vi "Actor Core.vi"(8 "error in":errorcluster, 11 "SPIController in":refnum<class "SPIController.lvclass">) -> (0 "error out":errorcluster, 3 "Actor out":refnum<class "Actor.lvclass">)   [LabVIEW 2023, in "SPIController.lvlib" / "SPIController.lvclass"]
doc: "(<B>Filename</B>: Actor Framework.lvlib:Actor.lvclass:Actor Core.vi)\n\nReceives messages to the actor, reacts to them, and initiates any error handling that may shut the actor down.\n\nDescendant classes may override this VI to append parallel tasks for the actor to complete while it handles messages. Overrides use the Call Parent Class Method node."
uses:
  SPIController.lvclass
  C:/Program Files/National Instruments/LabVIEW 2023/vi.lib/ActorFramework/Actor/Actor.lvclass
  <vilib>/ActorFramework/Actor/Actor.lvclass
  Controller_Cluster.ctl
  Controller_Scan_Cluster.ctl
  TranslationStage_UI/TranslationStage_UI/TranslationStageUI.lvclass
  <vilib>/ActorFramework/Message Enqueuer/Message Enqueuer.lvclass
  SinglePhotonInterferenceUI/SinglePhotonInterferenceUI/SinglePhotonInterferenceUI.lvclass
  <vilib>/ActorFramework/Actor/Actor.lvclass/Actor.ctl
  <vilib>/ActorFramework/Message Enqueuer/Message Enqueuer.lvclass/Message Enqueuer.ctl
  SPIController.lvclass/SPIController.ctl
  <vilib>/ActorFramework/Message Enqueuer/Init from Existing Queue.vi
  <vilib>/ActorFramework/Message Enqueuer/Enqueue.vi
  <vilib>/ActorFramework/Stop Msg/Stop Msg.lvclass
  C:/Program Files/National Instruments/LabVIEW 2023/vi.lib/ActorFramework/Message/Message.lvclass
  <vilib>/ActorFramework/Message Priority Queue/Priority Enqueue.vi
  SPIController.lvlib
  typedefs/typedefs.lvlib
panel:
  out "Multiharp Enqueuer":refnum<class "Message Enqueuer.lvclass">
  out "Translation Stage Enqueuer":refnum<class "Message Enqueuer.lvclass">
  out "Self Enqueuer":refnum<class "Message Enqueuer.lvclass">
  in  "TranslationStageUI.lvclass":refnum<class "TranslationStageUI.lvclass">
  in  "Ctrl Cluster":T1={"Actors Off"=FALSE, "Scan Cluster"={"Scan Segments X"=0, "Scan Segments Y"=0, "X Segments Left"=100, "Y Segments Left"=0, "Acq per step"=1, "X Home"=FALSE, "Y Home"=FALSE, "Axis"=enum."X", "Acquisitions Done"=0, "Get Measurements?"=FALSE}} {"Scan Cluster"."Scan Segments Y" max=100 step=1 scale=0.0..100.0; "Scan Cluster"."Acq per step" min=1 max=10000 step=1 scale=1.0..10000.0; "Scan Cluster"."Scan Segments X" max=100 step=1 scale=0.0..100.0}
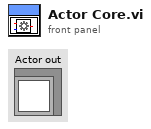
[diagram p1: front panel]
types:
  T1 = typedef "typedefs.lvlib/Controller_Cluster.ctl" = cluster{"Actors Off":bool, "Scan Cluster":T2}
  T2 = typedef "typedefs.lvlib/Controller_Scan_Cluster.ctl" = cluster{"Scan Segments X":u32, "Scan Segments Y":u32, "X Segments Left":u16, "Y Segments Left":u16, "Acq per step":u32, "X Home":bool, "Y Home":bool, "Axis":enum16{"X", "Y", "Z", "HOM"}, "Acquisitions Done":u16, "Get Measurements?":bool}
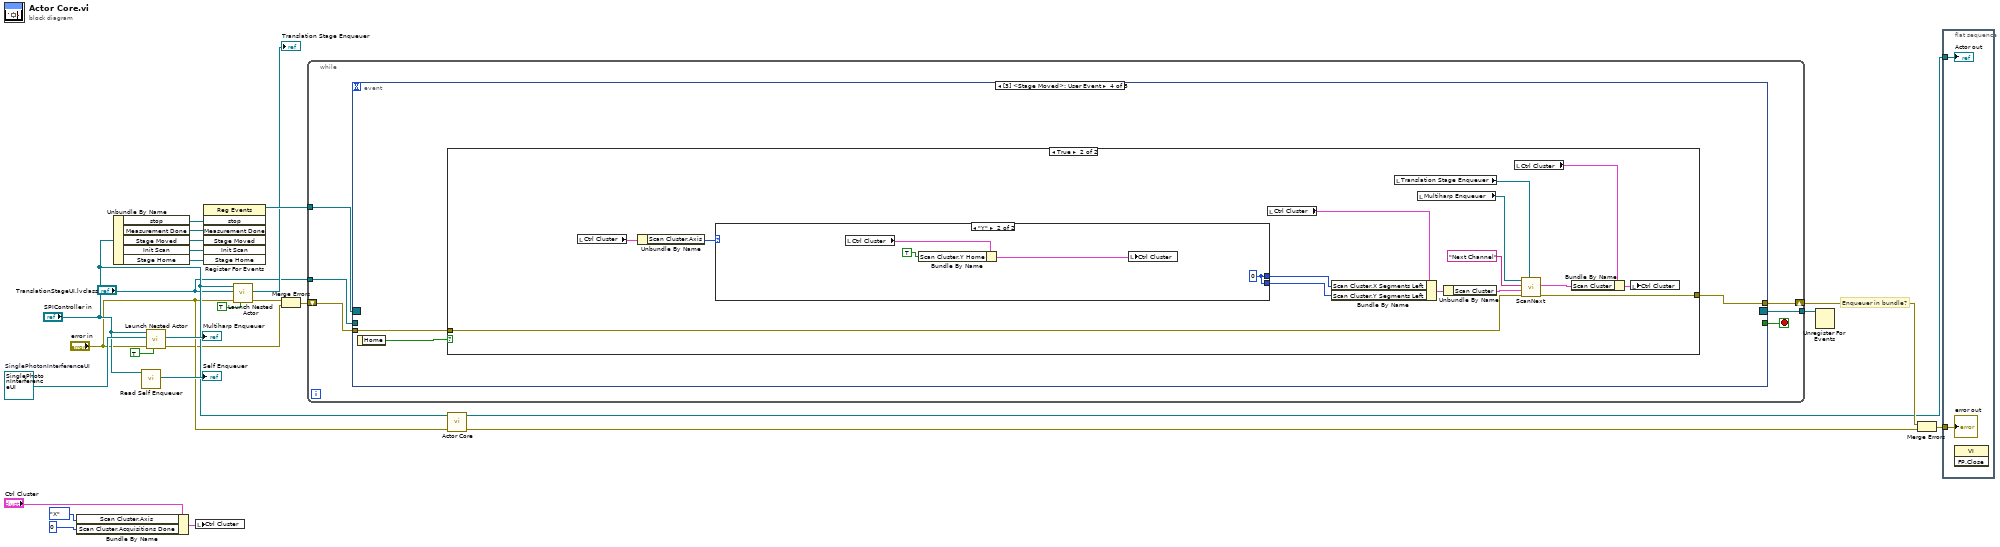
[diagram p0: block diagram]
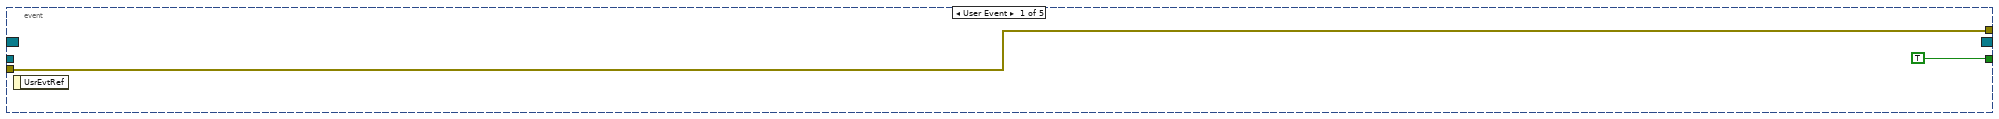
[diagram p2: hidden frame]
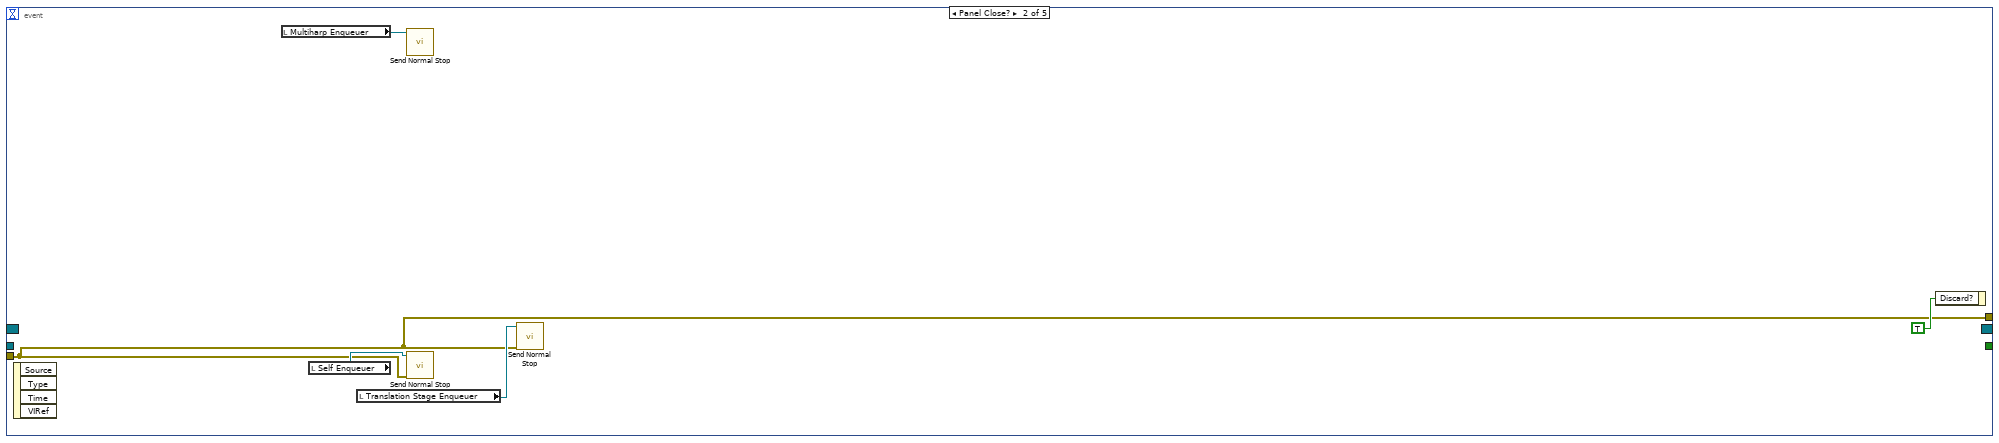
[diagram p3: hidden frame]
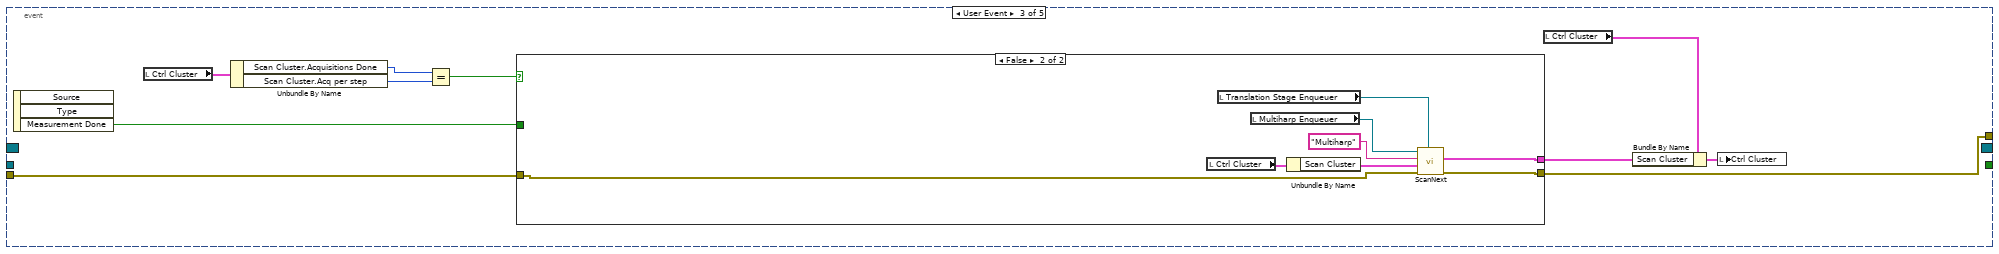
[diagram p4: hidden frame]
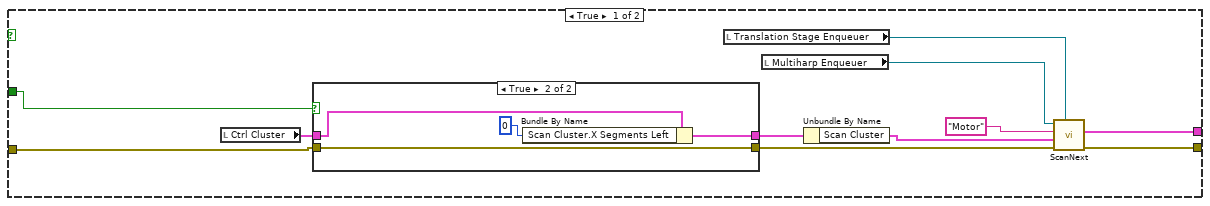
[diagram p5: hidden frame]
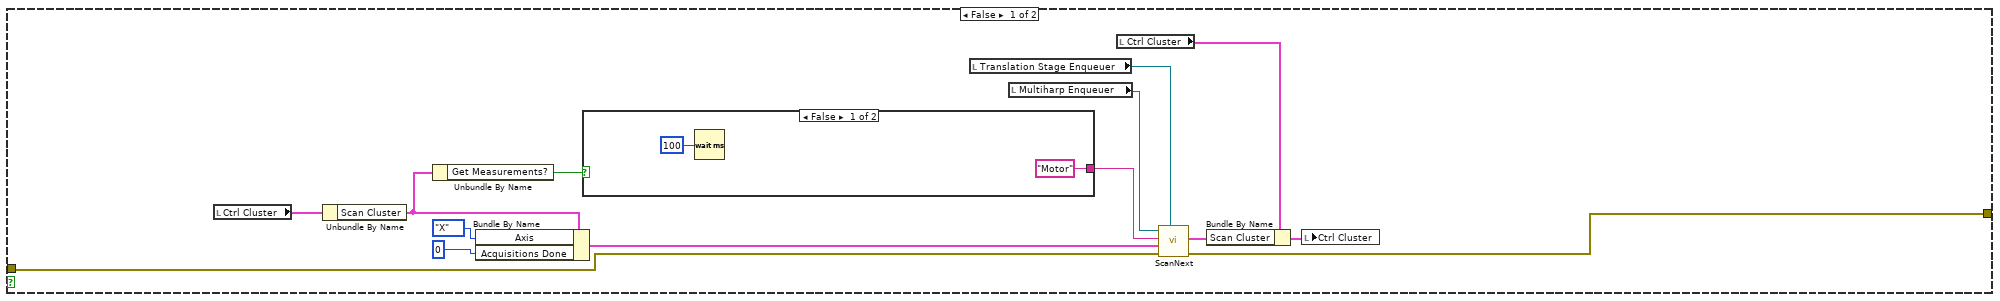
[diagram p7: hidden frame]
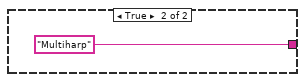
[diagram p8: hidden frame]
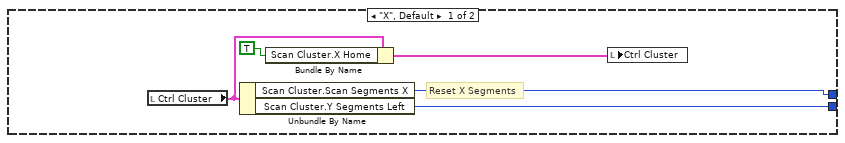
[diagram p9: hidden frame]
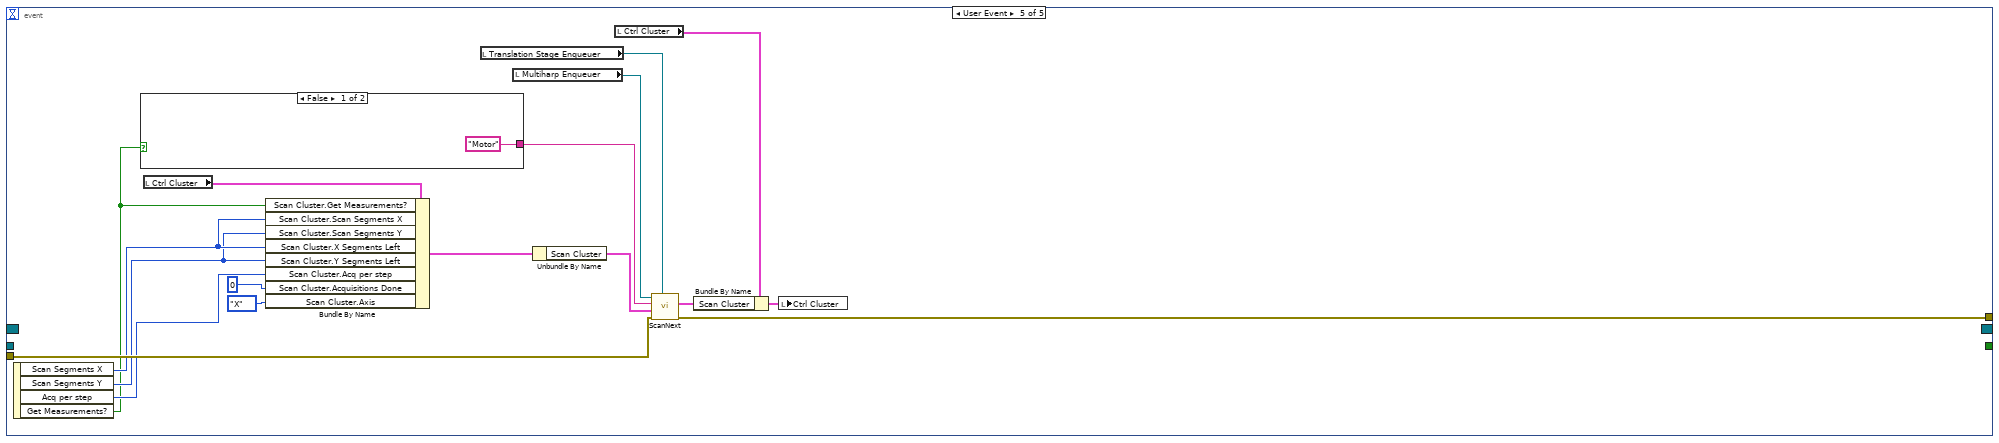
[diagram p10: hidden frame]
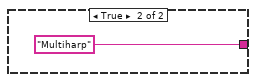
[diagram p11: hidden frame]
diagram:
  w27 = refnum<class "SinglePhotonInterferenceUI.lvclass"> refnum  # SinglePhotonInterferenceUI
  # "Enqueuer in bundle?"
  n1 = Bundle By Name(cluster="Ctrl Cluster", "Scan Cluster.Axis"=enum16{"X", "Y", "Z", "HOM"}."X", "Scan Cluster.Acquisitions Done"=u16 0) -> (w5:T1)
  n2 = Unbundle By Name("SPIController in") -> ("stop"=w24:refnum<user-event>, "Measurement Done"=w23:refnum<user-event>, "Stage Moved"=w15:refnum<user-event>, "Init Scan"=w14:refnum<user-event>, "Stage Home"=w13:refnum<user-event>)
  n3 = call <vilib>:"Read Self Enqueuer.vi"("Actor"="SPIController in") -> ("Self Enqueuer"=→"Self Enqueuer":refnum<class "Message Enqueuer.lvclass">)  [unwired: 10 in]
  n4 = call <vilib>:"Launch Nested Actor.vi"("Open Actor Core front panel? (F)"=TRUE, "error in (no error)"="error in", "Nested Actor"=w27, "Caller Actor in"="SPIController in") -> ("error out"=w6:errorcluster, "Nested Actor's Enqueuer"=→"Multiharp Enqueuer":refnum<class "Message Enqueuer.lvclass">)  [unwired: 5 in, 1 out]
  n5 = local write "Ctrl Cluster"(w5) -> ()
  n6 = register-events(w24, w23, w15, w14, w13) -> (reference out=w25:refnum<event-registration>)  [unwired: 2 in, 1 out]
  n7 = call <vilib>:"Launch Nested Actor.vi"("Open Actor Core front panel? (F)"=TRUE, "error in (no error)"="error in", "Nested Actor"="TranslationStageUI.lvclass", "Caller Actor in"="SPIController in") -> ("error out"=w7:errorcluster, "Nested Actor's Enqueuer"=→"Translation Stage Enqueuer":refnum<class "Message Enqueuer.lvclass">)  [unwired: 5 in, 1 out]
  n8 = Merge Errors(w7, w6) -> (w8:errorcluster)
  n9 = while {
    tunnel: w25 -> [w33]
    tunnel: [w31] -> w22
    shift-right: [w29] -> w19
    shift-left: w8 -> [w30]
    tunnel: "TranslationStageUI.lvclass" -> [w28]
    stop <- w32 stop-if-true
    n10 = event shown="[3] <Stage Moved>: User Event" {
      selector: w33 -> [_ _ _ _ _]
      dyn-events: [_ _ _ _ _] -> w31
      timeout: _ -> [_ _ _ _ _]
      tunnel: [TRUE _ _ _ _] -> w32
      tunnel: w30 -> [w34 w37 w50 w77 w134]
      tunnel: [w34 w37 w49 w78 w135] -> w29
      tunnel: w28 -> [_ _ _ _ _]
      event User Event {
        n11 = event-data() -> ()  [unwired: 1 in, 1 out]
      }
      event Panel Close? {
        n12 = event-data() -> ()  [unwired: 1 in, 4 out]
        n13 = local read "Multiharp Enqueuer"() -> (w36:refnum<class "Message Enqueuer.lvclass">)
        n14 = local read "Self Enqueuer"() -> (w39:refnum<class "Message Enqueuer.lvclass">)
        n15 = local read "Translation Stage Enqueuer"() -> (w38:refnum<class "Message Enqueuer.lvclass">)
        n16 = call <vilib>:"Send Normal Stop.vi"("Message Enqueuer"=w36) -> ()  [unwired: 10 in, 1 out]
        n17 = call <vilib>:"Send Normal Stop.vi"("error in (no error)"=w37, "Message Enqueuer"=w39) -> ()  [unwired: 9 in, 1 out]
        n18 = call <vilib>:"Send Normal Stop.vi"("error in (no error)"=w37, "Message Enqueuer"=w38) -> ()  [unwired: 9 in, 1 out]
        n19 = event-data("Discard?"=TRUE) -> ()  [unwired: 1 in, 1 out]
      }
      event User Event {
        n20 = event-data() -> ("Measurement Done"=w48:bool)  [unwired: 1 in, 2 out]
        n21 = local read "Ctrl Cluster"() -> (w43:T1)
        n22 = Unbundle By Name(w43) -> ("Scan Cluster.Acquisitions Done"=w45:u16, "Scan Cluster.Acq per step"=w46:u32)
        n23 = Equal?(x=w45, y=w46) -> (x = y?=w47:bool)
        n24 = case shown="False" w47 {
          tunnel: w50 -> [w51 w75]
          tunnel: [w61 w74] -> w49
          tunnel: w48 -> [w59 _]
          tunnel: [w58 w72] -> w44
          frame True {
            n25 = local read "Ctrl Cluster"() -> (w53:T1)
            n26 = case shown="True" w59 {
              tunnel: [w63 w66] -> w57
              tunnel: w53 -> [w63 w65]
              tunnel: [w62 w64] -> w52
              tunnel: w51 -> [w62 w64]
              frame False {
              }
              frame True {
                n27 = Bundle By Name(cluster=w65, "Scan Cluster.X Segments Left"=u16 0 ("Scanning Segments Left")) -> (w66:T1)
              }
            }
            n28 = local read "Translation Stage Enqueuer"() -> (w55:refnum<class "Message Enqueuer.lvclass">)
            n29 = local read "Multiharp Enqueuer"() -> (w56:refnum<class "Message Enqueuer.lvclass">)
            n30 = Unbundle By Name(w57) -> ("Scan Cluster"=w54:T2)
            n31 = call "ScanNext.vi"("Stage Enqueuer in"=w55, "error in"=w52, "Scan Cluster"=w54, "Instrument"="Motor", "MH Enqueuer in"=w56) -> ("error out"=w61:errorcluster, "Scan Cluster"=w58:T2)  [unwired: 5 in]
          }
          frame False {
            n32 = local read "Ctrl Cluster"() -> (w68:T1)
            n33 = local read "Translation Stage Enqueuer"() -> (w69:refnum<class "Message Enqueuer.lvclass">)
            n34 = local read "Multiharp Enqueuer"() -> (w70:refnum<class "Message Enqueuer.lvclass">)
            n35 = Unbundle By Name(w68) -> ("Scan Cluster"=w71:T2)
            n36 = call "ScanNext.vi"("Stage Enqueuer in"=w69, "error in"=w75, "Scan Cluster"=w71, "Instrument"="Multiharp", "MH Enqueuer in"=w70) -> ("error out"=w74:errorcluster, "Scan Cluster"=w72:T2)  [unwired: 5 in]
          }
        }
        n37 = local read "Ctrl Cluster"() -> (w42:T1)
        n38 = Bundle By Name(cluster=w42, "Scan Cluster"=w44) -> (w41:T1)
        n39 = local write "Ctrl Cluster"(w41) -> ()
      }
      event User Event {
        n40 = event-data() -> ("Home"=w76:bool)  [unwired: 1 in]
        n41 = case shown="True" w76 {
          tunnel: [w91 w102] -> w78
          tunnel: w77 -> [w90 w103]
          frame False {
            n42 = local read "Ctrl Cluster"() -> (w80:T1)
            n43 = Unbundle By Name(w80) -> ("Scan Cluster"=w86:T2)
            n44 = Unbundle By Name(w86) -> ("Get Measurements?"=w85:bool)
            n45 = Bundle By Name(cluster=w86, "Axis"=enum16{"X", "Y", "Z", "HOM"}."X", "Acquisitions Done"=u16 0) -> (w87:T2)
            n46 = case shown="False" w85 {
              tunnel: ["Motor" "Multiharp"] -> w92
              frame False {
                n47 = Wait (ms)(milliseconds to wait=u32 100) -> ()  [unwired: 1 out]
              }
              frame True {
              }
            }
            n48 = local read "Translation Stage Enqueuer"() -> (w82:refnum<class "Message Enqueuer.lvclass">)
            n49 = local read "Multiharp Enqueuer"() -> (w83:refnum<class "Message Enqueuer.lvclass">)
            n50 = local read "Ctrl Cluster"() -> (w79:T1)
            n51 = call "ScanNext.vi"("Stage Enqueuer in"=w82, "error in"=w90, "Scan Cluster"=w87, "Instrument"=w92, "MH Enqueuer in"=w83) -> ("error out"=w91:errorcluster, "Scan Cluster"=w89:T2)  [unwired: 5 in]
            n52 = Bundle By Name(cluster=w79, "Scan Cluster"=w89) -> (w81:T1)
            n53 = local write "Ctrl Cluster"(w81) -> ()
          }
          frame True {
            n54 = local read "Ctrl Cluster"() -> (w99:T1)
            n55 = Unbundle By Name(w99) -> ("Scan Cluster.Axis"=w104:enum16{"X", "Y", "Z", "HOM"})
            n56 = case shown="\"Y\"" w104 {
              tunnel: [w115 w118] -> w107
              tunnel: [w114 w118] -> w106
              frame "X", Default {
                # "Reset X Segments"
                n57 = local read "Ctrl Cluster"() -> (w112:T1)
                n58 = Unbundle By Name(w112) -> ("Scan Cluster.Scan Segments X"=w115:u32, "Scan Cluster.Y Segments Left"=w114:u16)
                n59 = Bundle By Name(cluster=w112, "Scan Cluster.X Home"=TRUE ("Scan Cluster.Y Home")) -> (w111:T1)
                n60 = local write "Ctrl Cluster"(w111) -> ()
              }
              frame "Y" {
                w118 = u32 0 ("Scan Segments X")
                n61 = local read "Ctrl Cluster"() -> (w117:T1)
                n62 = Bundle By Name(cluster=w117, "Scan Cluster.Y Home"=TRUE) -> (w116:T1)
                n63 = local write "Ctrl Cluster"(w116) -> ()
              }
            }
            n64 = local read "Ctrl Cluster"() -> (w98:T1)
            n65 = Bundle By Name(cluster=w98, "Scan Cluster.X Segments Left"=w107, "Scan Cluster.Y Segments Left"=w106) -> (w110:T1)
            n66 = local read "Translation Stage Enqueuer"() -> (w100:refnum<class "Message Enqueuer.lvclass">)
            n67 = local read "Multiharp Enqueuer"() -> (w101:refnum<class "Message Enqueuer.lvclass">)
            n68 = Unbundle By Name(w110) -> ("Scan Cluster"=w109:T2)
            n69 = local read "Ctrl Cluster"() -> (w97:T1)
            n70 = call "ScanNext.vi"("Stage Enqueuer in"=w100, "error in"=w103, "Scan Cluster"=w109, "Instrument"="Next Channel", "MH Enqueuer in"=w101) -> ("error out"=w102:errorcluster, "Scan Cluster"=w108:T2)  [unwired: 5 in]
            n71 = Bundle By Name(cluster=w97, "Scan Cluster"=w108) -> (w96:T1)
            n72 = local write "Ctrl Cluster"(w96) -> ()
          }
        }
      }
      event User Event {
        n73 = event-data() -> ("Scan Segments X"=w132:u32, "Scan Segments Y"=w129:u32, "Acq per step"=w128:u8, "Get Measurements?"=w126:bool)  [unwired: 1 in]
        n74 = case shown="False" w126 {
          tunnel: ["Motor" "Multiharp"] -> w136
          frame False {
          }
          frame True {
          }
        }
        n75 = local read "Ctrl Cluster"() -> (w122:T1)
        n76 = Bundle By Name(cluster=w122, "Scan Cluster.Get Measurements?"=w126, "Scan Cluster.Scan Segments X"=w132, "Scan Cluster.Scan Segments Y"=w129, "Scan Cluster.X Segments Left"=w132, "Scan Cluster.Y Segments Left"=w129, "Scan Cluster.Acq per step"=w128, "Scan Cluster.Acquisitions Done"=u16 0, "Scan Cluster.Axis"=enum16{"X", "Y", "Z", "HOM"}."X") -> (w133:T1)
        n77 = local read "Translation Stage Enqueuer"() -> (w123:refnum<class "Message Enqueuer.lvclass">)
        n78 = local read "Multiharp Enqueuer"() -> (w124:refnum<class "Message Enqueuer.lvclass">)
        n79 = Unbundle By Name(w133) -> ("Scan Cluster"=w131:T2)
        n80 = local read "Ctrl Cluster"() -> (w121:T1)
        n81 = call "ScanNext.vi"("Stage Enqueuer in"=w123, "error in"=w134, "Scan Cluster"=w131, "Instrument"=w136, "MH Enqueuer in"=w124) -> ("error out"=w135:errorcluster, "Scan Cluster"=w130:T2)  [unwired: 5 in]
        n82 = Bundle By Name(cluster=w121, "Scan Cluster"=w130) -> (w120:T1)
        n83 = local write "Ctrl Cluster"(w120) -> ()
      }
    }
  }
  n84 = call-parent "Actor Core.vi"("error in"="error in", "Actor in"="SPIController in") -> ("error out"=w2:errorcluster, "Actor out"=w4:refnum<class "Actor.lvclass">)  [unwired: 8 in]
  n85 = Unregister For Events(event registration refnum=w22) -> ()  [unwired: 1 in, 1 out]
  n86 = Merge Errors(w19, w2) -> (w3:errorcluster)
  n87 = flat-sequence {
    tunnel: w4 -> [w140]
    tunnel: w3 -> [w139]
    frame #0 {
      n88 = invoke class="VI" method="FP.Close"() -> ()  [unwired: 3 in, 3 out]
      "Actor out" <- w140
      "error out" <- w139
    }
  }
